vi "Send Message to Python.vi"(7 "Server Alias":string, 8 "error in (no error)":errorcluster, 11 "Message":T1={"Command"="zxcvbnm,", "Data"=["asdfghjk", "qwertyui"], "Script ID"=0, "LabVIEW Server ID"="zxcvbnm,", "Python Message ID"=0}) -> (0 "error out":errorcluster)   [LabVIEW 2013, in "TS.lvlib"]
doc: "This VI pushes a message onto the LvPy queue so that the Server.vi can send it to Python."
uses:
  TS.lvlib
  LabVIEW Python Connector Message.ctl
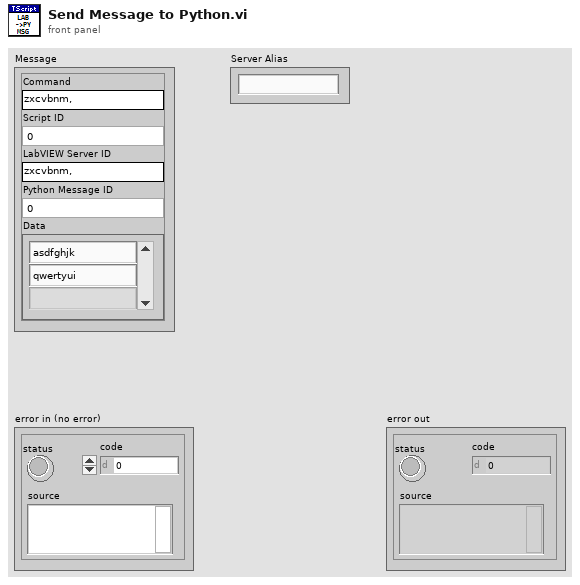
[diagram p1: front panel]
types:
  T1 = typedef "TS.lvlib/LabVIEW Python Connector Message.ctl" = cluster{"Command":string, "Data":string[], "Script ID":i64, "LabVIEW Server ID":string, "Python Message ID":i32}
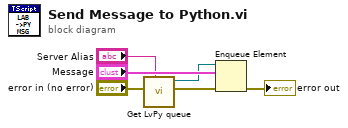
[diagram p0: block diagram]
diagram:
  n1 = call "Get LvPy queue.vi"("Server Alias"="Server Alias", "Error In"="error in (no error)") -> ("Error Out"=w3:errorcluster, "LvPy queue"=w2:refnum<queue>)  [unwired: 8 in]
  n2 = Enqueue Element(queue=w2, element="Message", error in (no error)=w3) -> (error out=→"error out":errorcluster)  [unwired: 1 in, 2 out]
